vi "Arm Command.vi"(4 "Controller name":string, 7 "Objects enqueuers":refnum<class "Message Enqueuer.lvclass">[](array[class]), 8 "error in (no error)":errorcluster, 9 "Request type":T1, 10 "Objects":string[](array[string]), 11 "Pulse Controller in":refnum<class "Pulse Controller.lvclass">) -> (0 "error out":errorcluster, 3 "Pulse Controller out":refnum<class "Pulse Controller.lvclass">)   [LabVIEW 2024, in "Pulse Controller.lvclass"]
uses:
  Pulse Controller.lvclass
  C:/Git/LabActor/Worker/Worker Actor/Worker Actor.lvclass
  C:/Git/LabActor/Controllers/Process Controller/Process Controller.lvclass
  C:/Git/LabActor/Template Module/Template Module.lvclass
  C:/Program Files/National Instruments/LabVIEW 2024/vi.lib/ActorFramework/Actor/Actor.lvclass
  <vilib>/ActorFramework/Message Enqueuer/Message Enqueuer.lvclass
  Process Controller/Request type.ctl
  Worker/Worker Actor/Worker Actor.lvclass/Worker Actor.ctl
  NHMFL_Core/Libraries/Instruments/Instrument Driver/Worker State.ctl
  Publish-Subscribe/Context.ctl
  Process Controller/Process Controller.lvclass/Process Controller.ctl
  Template Module/Template Module.lvclass/Template Module.ctl
  Pulse Controller.lvclass/Pulse Controller.ctl
  <vilib>/ActorFramework/Actor/Actor.lvclass/Actor.ctl
  <vilib>/ActorFramework/Message Enqueuer/Message Enqueuer.lvclass/Message Enqueuer.ctl
  Publish-Subscribe/Interfaces/Publisher Messages/Subscribe Msg/Subscribe Msg.lvclass/Subscribe Msg.ctl
  Template Module Messages/Write tdms stream Msg/Write tdms stream Msg.lvclass/Write tdms stream Msg.ctl
  Pulse Recorders/Interfaces/Pulse Recorder Messages/Arm Msg/Arm Msg.lvclass/Arm Msg.ctl
  Process Controller/Write Active measurements enqueuers.vi
  Process Controller/Write Active measurements names.vi
  Template Module/Read Name.vi
  Template Module/Write State.vi
  Template Module/Read State.vi
  <vilib>/ActorFramework/Message Enqueuer/Init from Existing Queue.vi
  <vilib>/ActorFramework/Message Enqueuer/Enqueue.vi
  Publish-Subscribe/Interfaces/Publisher Messages/Subscribe Msg/Subscribe Msg.lvclass
  C:/Program Files/National Instruments/LabVIEW 2024/vi.lib/ActorFramework/Message/Message.lvclass
  Template Module Messages/Write tdms stream Msg/Write tdms stream Msg.lvclass
  Pulse Recorders/Interfaces/Pulse Recorder Messages/Arm Msg/Arm Msg.lvclass
  <vilib>/ActorFramework/Message Priority Queue/Priority Enqueue.vi
  Measurements/Response Synchronizer/Response Synchronizer.lvclass
  <vilib>/ActorFramework/Actor/Actor.lvclass
  C:/Git/LabActor/Worker/Woker Interface/Worker.lvclass
  C:/Git/LabActor/Publish-Subscribe/Interfaces/Subscriber/Subscriber.lvclass
  C:/Git/LabActor/Controllers/Pulse Controller/Pulse Controller.lvclass
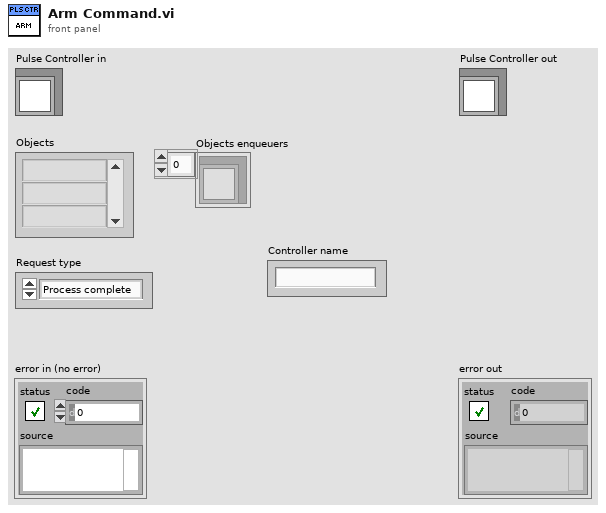
[diagram p1: front panel]
types:
  T1 = typedef "Request type.ctl" = enum16{"Process complete", "User command", "Auto-restart", "Error"}
  T2 = typedef "Context.ctl" = cluster{"Topic":string, "Source":string}
  T3 = typedef "Worker State.ctl" = enum16{"Idle", "Starting", "Working", "Stopping"}
  T4 = typedef "Pulse Controller Configuration.ctl" = cluster{"Pre-trigger duration":dbl, "Post-trigger duration":dbl, "Open plot after pulse":bool, "Auto-rearm":bool, "Back-up raw data":bool, "File prefix":string}
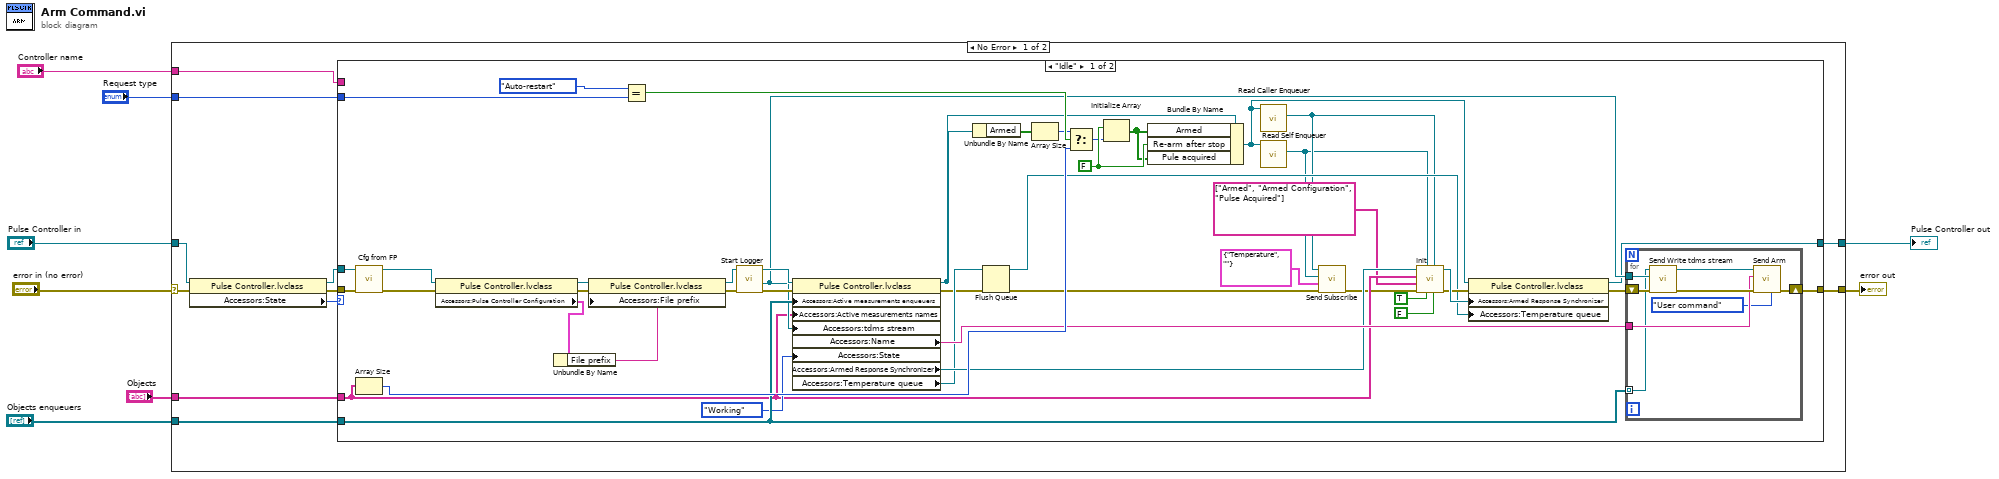
[diagram p0: block diagram]
diagram:
  n1 = case shown="No Error" "error in (no error)" {
    selector: "error in (no error)" -> [w15 w76]
    tunnel: [w16 w76] -> w7
    tunnel: [w9 w75] -> w5
    tunnel: "Pulse Controller in" -> [w14 w75]
    tunnel: "Objects" -> [w13 _]
    tunnel: "Controller name" -> [w12 _]
    tunnel: "Objects enqueuers" -> [w11 _]
    tunnel: "Request type" -> [w10 _]
    frame No Error {
      n2 = property class="Pulse Controller.lvclass"(reference=w14, error in=w15) -> (reference out=w18:refnum<class "Pulse Controller.lvclass">, error out=w19:errorcluster, "Accessors:State"=w17:T3)
      n3 = case shown="\"Idle\"" w17 {
        tunnel: [w48 w74] -> w16
        tunnel: [w35 w73] -> w9
        tunnel: w11 -> [w50 _]
        tunnel: w19 -> [w54 w74]
        tunnel: w13 -> [w42 _]
        tunnel: w18 -> [w55 w73]
        tunnel: w10 -> [w63 _]
        tunnel: w12 -> [_ _]
        frame "Idle" {
          w64 = FALSE
          n4 = call-dynamic "Cfg from FP.vi"("error in (no error)"=w54, "Measure Object in"=w55) -> ("error out"=w53:errorcluster, "Measure Object out"=w25:refnum<class "Pulse Controller.lvclass">)  [unwired: 8 in]
          n5 = Array Size(array=w42) -> (size(s)=w59:i32)
          n6 = property class="Pulse Controller.lvclass"(reference=w25, error in=w53) -> (reference out=w23:refnum<class "Pulse Controller.lvclass">, error out=w26:errorcluster, "Accessors:Pulse Controller Configuration"=w21:T4)
          n7 = Unbundle By Name(w21) -> ("File prefix"=w20:string)
          n8 = property class="Pulse Controller.lvclass"(reference=w23, error in=w26, "Accessors:File prefix"=w20) -> (reference out=w22:refnum<class "Pulse Controller.lvclass">, error out=w24:errorcluster)
          n9 = Equal?(x=Request_type."Auto-restart", y=w63) -> (x = y?=w60:bool)
          n10 = call-dynamic "Start Logger.vi"("error in (no error)"=w24, "Worker in"=w22) -> ("error out"=w52:errorcluster, "tdms stream out"=w49:refnum<k34>, "Worker out"=w51:refnum<class "Pulse Controller.lvclass">)  [unwired: 6 in, 1 out]
          n11 = property class="Pulse Controller.lvclass"(reference=w51, error in=w52, "Accessors:Active measurements enqueuers"=w50, "Accessors:Active measurements names"=w42, "Accessors:tdms stream"=w49, "Accessors:State"=Worker_State."Working" ("State")) -> (reference out=w38:refnum<class "Pulse Controller.lvclass">, error out=w32:errorcluster, "Accessors:Name"=w47:string, "Accessors:Armed Response Synchronizer"=w45:refnum<class "Response Synchronizer.lvclass">, "Accessors:Temperature queue"=w34:refnum<queue>)
          n12 = Unbundle By Name(w38) -> ("Armed"=w61:bool[])
          n13 = Flush Queue(queue=w34, error in (no error)=w32) -> (queue out=w33:refnum<queue>, error out=w28:errorcluster)  [unwired: 1 out]
          n14 = Array Size(array=w61) -> (size(s)=w58:i32)
          n15 = Select(t=w58, s=w60, f=w59) -> (s? t:f=w57:i32)
          n16 = Initialize Array(w64, w57) -> (w56:bool[])
          n17 = Bundle By Name(cluster=w38, "Armed"=w56, "Re-arm after stop"=w64, "Pule acquired"=w56) -> (w37:refnum<class "Pulse Controller.lvclass">)
          n18 = call <vilib>:"Read Caller Enqueuer.vi"("Actor"=w37) -> ("Caller Enqueuer"=w31:refnum<class "Message Enqueuer.lvclass">)  [unwired: 10 in]
          n19 = call <vilib>:"Read Self Enqueuer.vi"("Actor"=w37) -> ("Self Enqueuer"=w30:refnum<class "Message Enqueuer.lvclass">)  [unwired: 10 in]
          n20 = call "Send Subscribe.vi"("error in (no error)"=w28, "Context"=T2 {"Topic"="Temperature", "Source"=""}, "Subscriber Enq"=w30, "Message Enqueuer"=w31) -> ("error out"=w27:errorcluster)  [unwired: 6 in, 1 out]
          n21 = call-dynamic "Init.vi"("Pre-preocess datasockets"=FALSE, "Caller Enqueuer"=w31, "Subscribe"=TRUE, "Self Enqueuer"=w30, "error in (no error)"=w27, "Topics"=string[] ["Armed", "Armed Configuration", "Pulse Acquired"], "Responder names"=w42, "Response Synchronizer in"=w45) -> ("error out"=w43:errorcluster, "Response Synchronizer out"=w44:refnum<class "Response Synchronizer.lvclass">)  [unwired: 1 in, 1 out]
          n22 = property class="Pulse Controller.lvclass"(reference=w37, error in=w43, "Accessors:Armed Response Synchronizer"=w44, "Accessors:Temperature queue"=w33) -> (reference out=w35:refnum<class "Pulse Controller.lvclass">, error out=w36:errorcluster)
          n23 = for {
            shift-right: [w68] -> w48
            shift-left: w36 -> [w72]
            tunnel: w50 -> [w65] mode=indexing
            tunnel: w49 -> [w71]
            tunnel: w47 -> [w69]
            n24 = call "Send Write tdms stream.vi"("error in (no error)"=w72, "tdms stream"=w71, "Message Enqueuer"=w65) -> ("error out"=w70:errorcluster, "Message Enqueuer out"=w66:refnum<class "Message Enqueuer.lvclass">)  [unwired: 7 in]
            n25 = call "Send Arm.vi"("Request type"=Request_type."User command", "error in (no error)"=w70, "Requester"=w69, "Message Enqueuer"=w66) -> ("error out"=w68:errorcluster)  [unwired: 6 in, 1 out]
          }
        }
        frame "Working", Default {
        }
      }
    }
    frame Error {
    }
  }
  "error out" <- w7
  "Pulse Controller out" <- w5
